vi "Modbus Samsung Mod.vi"(5 "address":string, 6 "# Racks":i32=1, 7 "port (502)":u16=502, 8 "Error In":errorcluster, 10 "ES Reset":bool=TRUE, 11 "ES ON Array":bool[](array[boolean])) -> (0 "Error Out":errorcluster, 1 "Current Limit Parameters Out":T5 {"Min Cell Voltage Actual Value" format="%#.2f"; "Max Cell Voltage Actual Value" format="%#.2f"}, 2 "Energy Storage String Data Out":T3, 3 "Energy Storage System Data Out":T1={"Voltage"=0.0, "Current"=0.0, "SOC Avg"=0.0, "Faults"=0, "Alarms"=0, "# Strings"=0, "Max Temp"=0, "Min Temp"=0, "Max Cell Voltage"=0.0, "Min Cell Voltage"=0.0, "Energy Capacity"=0.0, "Energy Remaining"=0.0, "SOC Min"=0.0, "SOC Max"=0.0, "ES Fault"=FALSE, "String Select"=enum."3 Strings", "ES Com Fault"=FALSE, "SOH Avg"=0.0}, 4 "Contactor CMD FB":bool[](array[boolean]))   [LabVIEW 2014]
uses:
  Controls/Current Limit Parameters.ctl
  Controls/ES String Array.ctl
  Controls/ES String Data.ctl
  Controls/ES System Data.ctl
  Controls/StringSelector.ctl
  Controls/ModbusState.ctl
  <vilib>/Modbus/master/Modbus Master.lvclass
  <vilib>/Modbus/master/Create Master Instance (TCP).vi
panel:
  out "Error Count":i32
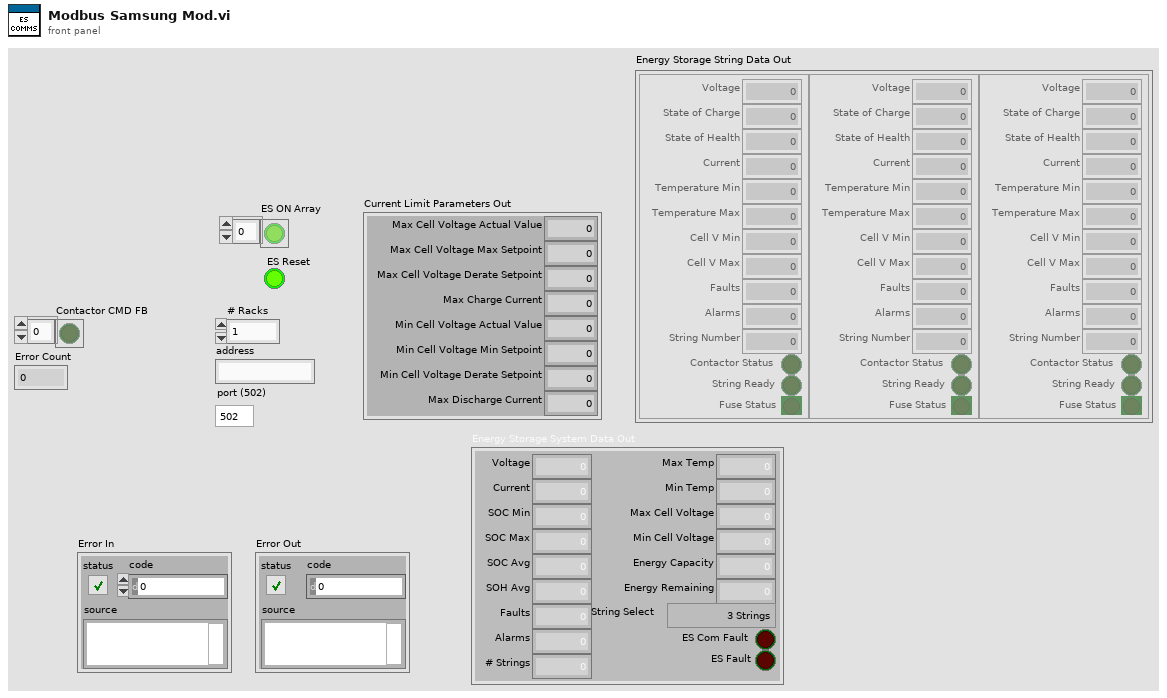
[diagram p1: front panel]
types:
  T1 = typedef "ES System Data.ctl" = cluster{"Voltage":sgl, "Current":sgl, "SOC Avg":sgl, "Faults":u16, "Alarms":u16, "# Strings":u16, "Max Temp":i16, "Min Temp":i16, "Max Cell Voltage":sgl, "Min Cell Voltage":sgl, "Energy Capacity":sgl, "Energy Remaining":sgl, "SOC Min":sgl, "SOC Max":sgl, "ES Fault":bool, "String Select":T2, "ES Com Fault":bool, "SOH Avg":sgl}
  T2 = typedef "StringSelector.ctl" = enum16{"1 String (1)", "1 String (2)", "1 String (3)", "2 Strings (1 2)", "2 Strings (2 3)", "2 Strings (1 3)", "3 Strings"}
  T3 = typedef "ES String Array.ctl" = T4[]
  T4 = typedef "ES String Data.ctl" = cluster{"Voltage":sgl, "State of Charge":sgl, "Current":sgl, "Temperature Min":i16, "Temperature Max":i16, "Faults":u16, "Alarms":u16, "String Number":u16, "Contactor Status":bool, "String Ready":bool, "Fuse Status":bool, "Cell V Max":dbl, "Cell V Min":dbl, "State of Health":sgl}
  T5 = typedef "Current Limit Parameters.ctl" = cluster{"Max Cell Voltage Max Setpoint":dbl, "Max Cell Voltage Actual Value":dbl, "Max Cell Voltage Derate Setpoint":dbl, "Max Charge Current":dbl, "Min Cell Voltage Min Setpoint":dbl, "Min Cell Voltage Actual Value":dbl, "Min Cell Voltage Derate Setpoint":dbl, "Max Discharge Current":dbl}
  T6 = typedef "ModbusState.ctl" = enum16{"Connect", "Disconnect", "Set Basic Objects", "Get Basic Objects", "Read", "Write", "Read/Write"}
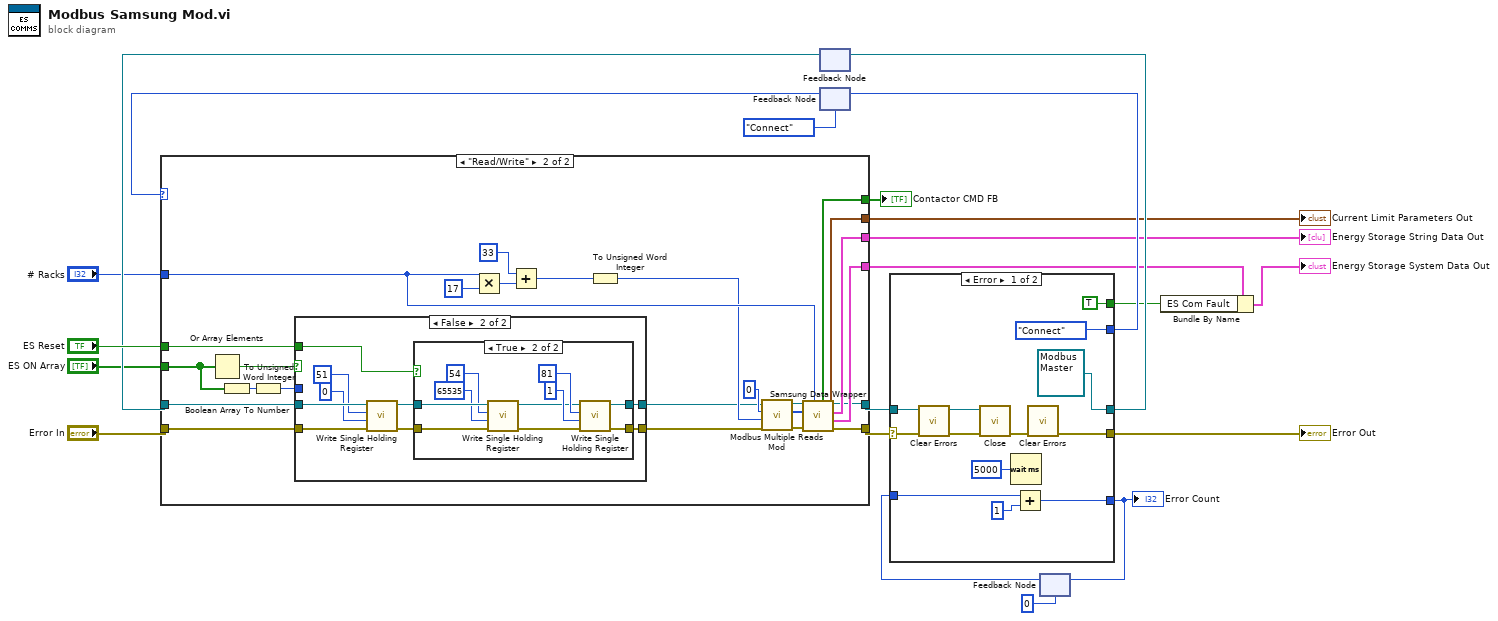
[diagram p0: block diagram]
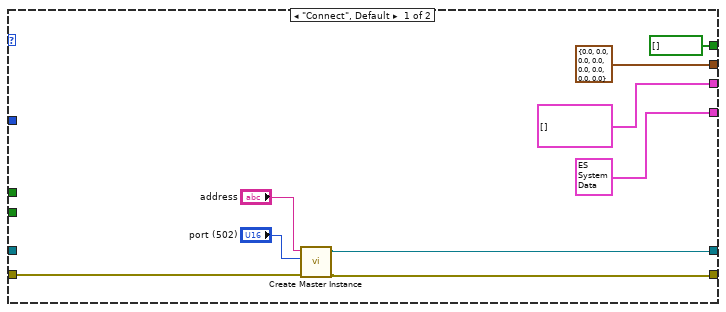
[diagram p2: hidden frame]
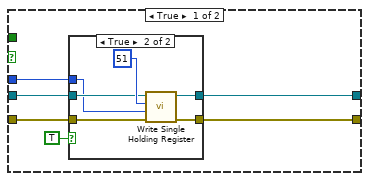
[diagram p3: hidden frame]
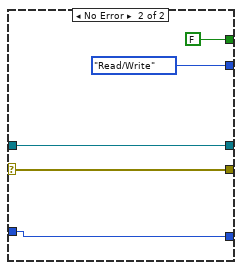
[diagram p6: hidden frame]
diagram:
  n1 = feedback #1() -> (w17:refnum<class "Modbus Master.lvclass">)  [unwired: 1 in]
  n2 = feedback #2(ModbusState."Connect" ("Modbus State In")) -> (w18:T6)
  n3 = case shown="\"Read/Write\"" w18 {
    tunnel: "Error In" -> [w30 w53]
    tunnel: [w22 w37] -> w13
    tunnel: w17 -> [_ w52]
    tunnel: [w23 w54] -> w15
    tunnel: "ES Reset" -> [_ w51]
    tunnel: "ES ON Array" -> [_ w49]
    tunnel: "# Racks" -> [_ w42]
    tunnel: [T5 {"Max Cell Voltage Max Setpoint"=0.0, "Max Cell Voltage Actual Value"=0.0, "Max Cell Voltage Derate Setpoint"=0.0, "Max Charge Current"=0.0, "Min Cell Voltage Min Setpoint"=0.0, "Min Cell Voltage Actual Value"=0.0, "Min Cell Voltage Derate Setpoint"=0.0, "Max Discharge Current"=0.0} ("Current Limit Parameters Out") w41] -> w10
    tunnel: [T3 [] ("Energy Storage String Data Out") w40] -> w9
    tunnel: [T1 {"Voltage"=0.0, "Current"=0.0, "SOC Avg"=0.0, "Faults"=0, "Alarms"=0, "# Strings"=0, "Max Temp"=0, "Min Temp"=0, "Max Cell Voltage"=0.0, "Min Cell Voltage"=0.0, "Energy Capacity"=0.0, "Energy Remaining"=0.0, "SOC Min"=0.0, "SOC Max"=0.0, "ES Fault"=FALSE, "String Select"=enum."3 Strings", "ES Com Fault"=TRUE, "SOH Avg"=0.0} ("Energy Storage System Data Out") w39] -> w8
    tunnel: [bool[] [] ("Contactor CMD") w33] -> w5
    frame "Connect", Default {
      n4 = call-poly <vilib>:"Create Master Instance.vi"("error in (no error)"=w30, "port (502)"="port (502)", "address"="address") -> ("error out"=w23:errorcluster, "TCP master instance"=w22:refnum<class "Modbus Master.lvclass">)  [unwired: 7 in]
    }
    frame "Read/Write" {
      n5 = Or Array Elements(Boolean array=w49) -> (logical OR=w50:bool)
      n6 = Boolean Array To Number(Boolean array=w49) -> (number=w48:u32)
      n7 = To Unsigned Word Integer(number=w48) -> (unsigned 16bit integer=w47:u16)
      n8 = case shown="False" w50 {
        tunnel: w53 -> [w60 w74]
        tunnel: w52 -> [w57 w72]
        tunnel: w51 -> [_ w77]
        tunnel: [w59 w76] -> w32
        tunnel: [w58 w75] -> w31
        tunnel: w47 -> [w56 _]
        frame True {
          n9 = case shown="True" TRUE {
            tunnel: w60 -> [w61 w67]
            tunnel: [w61 w66] -> w59
            tunnel: [w62 w65] -> w58
            tunnel: w57 -> [w62 w64]
            tunnel: w56 -> [_ w63]
            frame False {
            }
            frame True {
              n10 = call-dynamic "Write Single Holding Register.vi"("error in (no error)"=w67, "holding register value"=w63, "address"=u16 51, "Modbus master in"=w64) -> ("error out"=w66:errorcluster, "Modbus master out"=w65:refnum<class "Modbus Master.lvclass">)  [unwired: 6 in]
            }
          }
        }
        frame False {
          n11 = call-dynamic "Write Single Holding Register.vi"("error in (no error)"=w74, "holding register value"=u16 0, "address"=u16 51, "Modbus master in"=w72) -> ("error out"=w73:errorcluster, "Modbus master out"=w71:refnum<class "Modbus Master.lvclass">)  [unwired: 6 in]
          n12 = case shown="True" w77 {
            tunnel: w73 -> [w79 w89]
            tunnel: w71 -> [w78 w88]
            tunnel: [w79 w82] -> w76
            tunnel: [w78 w80] -> w75
            frame False {
            }
            frame True {
              n13 = call-dynamic "Write Single Holding Register.vi"("error in (no error)"=w89, "holding register value"=u16 65535, "address"=u16 54, "Modbus master in"=w88) -> ("error out"=w83:errorcluster, "Modbus master out"=w81:refnum<class "Modbus Master.lvclass">)  [unwired: 6 in]
              n14 = call-dynamic "Write Single Holding Register.vi"("error in (no error)"=w83, "holding register value"=u16 1, "address"=u16 81, "Modbus master in"=w81) -> ("error out"=w82:errorcluster, "Modbus master out"=w80:refnum<class "Modbus Master.lvclass">)  [unwired: 6 in]
            }
          }
        }
      }
      n15 = Multiply(x=w42, y=u8 17) -> (x*y=w45:i32)
      n16 = Add(x=u8 33, y=w45) -> (x+y=w43:i32)
      n17 = To Unsigned Word Integer(number=w43) -> (unsigned 16bit integer=w35:u16)
      n18 = call "Modbus Multiple Reads Mod.vi"("Error In"=w32, "# elements to read"=w35, "Starting Address"=u16 0 ("starting address"), "Modbus Master In"=w31) -> ("Error Out"=w36:errorcluster, "register values"=w38:u16[], "Modbus Master Out"=w37:refnum<class "Modbus Master.lvclass">)  [unwired: 5 in]
      n19 = call "Samsung Data Wrapper.vi"("# Racks"=w42, "Error In"=w36, "Samsung Data In"=w38) -> ("Error Out"=w54:errorcluster, "Energy Storage System Data Out"=w39:T1, "Energy Storage String Data Out"=w40:T3, "Current Limit Parameters Out"=w41:T5, "Contactor CMD"=w33:bool[])  [unwired: 4 in]
    }
  }
  "Current Limit Parameters Out" <- w10
  "Energy Storage String Data Out" <- w9
  "Contactor CMD FB" <- w5
  n20 = feedback #3(0) -> (w4:i32)
  n21 = case shown="Error" w15 {
    selector: w15 -> [w91 w106]
    tunnel: w13 -> [w99 w105]
    tunnel: [w100 w106] -> w14
    tunnel: [refnum<class "Modbus Master.lvclass"> refnum ("TCP master instance") w105] -> w12
    tunnel: [ModbusState."Connect" ("Modbus State In") ModbusState."Read/Write" ("Modbus State In")] -> w11
    tunnel: [TRUE FALSE] -> w6
    tunnel: w4 -> [w95 w102]
    tunnel: [w94 w102] -> w2
    frame Error {
      n22 = call <vilib>:"Clear Errors.vi"("error in (no error)"=w91) -> ("error out"=w90:errorcluster)  [unwired: 5 in, 1 out]
      n23 = call-dynamic "Close.vi"("error in (no error)"=w90, "Modbus master in"=w99) -> ("error out"=w101:errorcluster)  [unwired: 9 in]
      n24 = Wait (ms)(milliseconds to wait=u32 5000) -> ()  [unwired: 1 out]
      n25 = Add(x=w95, y=1) -> (x+y=w94:i32)
      n26 = call <vilib>:"Clear Errors.vi"("error in (no error)"=w101) -> ("error out"=w100:errorcluster)  [unwired: 5 in, 1 out]
    }
    frame No Error {
    }
  }
  "Error Out" <- w14
  "Error Count" <- w2
  n27 = feedback-in #1(w12) -> ()
  n28 = feedback-in #2(w11) -> ()
  n29 = feedback-in #3(w2) -> ()
  n30 = Bundle By Name(cluster=w8, "ES Com Fault"=w6) -> (→"Energy Storage System Data Out":T1)
